vi "Spot Chessboard AR.vi"() -> ()   [LabVIEW 2020]
uses:
  g_ar_toolkit.feature_detection/Chessboard Corner Info.ctl
  g_ar_toolkit.common/Object Point (Float).ctl
  g_ar_toolkit.ar/Camera Parameters.ctl
  g_ar_toolkit.ar/Camera Matrix.ctl
  g_ar_toolkit.ar/Camera Distortion Coefficients.ctl
  g_ar_toolkit.common/Image Size (Integer).ctl
  g_ar_toolkit.ar/Point Correspondence Set.ctl
  g_ar_toolkit.common/Image Point (Float).ctl
  g_ar_toolkit.image/Image Read Size.ctl
  g_ar_toolkit.image/CreateEmptyImageGreyscale.vi
  g_ar_toolkit.image/CreateEmptyImageARGB.vi
  g_ar_toolkit.image/ReadImageFileARGB.vi
  g_ar_toolkit.feature_detection/FindChessboardCornersGreyscale.vi
  g_ar_toolkit.ar/SolvePnP-Iterative.vi
  g_ar_toolkit.image/CopyPixmapToImageFlattenMaskARGB.vi
  g_ar_toolkit.image/MaskFromColour.vi
  g_ar_toolkit.image/BitwiseNOTGreyscale.vi
  g_ar_toolkit.image/InsertImageGreyscaleMaskARGB.vi
  g_ar_toolkit.image/DrawImageToPictureGreyscale.vi
  g_ar_toolkit.image/DrawImageToPictureARGB.vi
  g_ar_toolkit.ar/Create Mesh form Verticies.vi
  g_ar_toolkit.ar/Apply Material Information.vi
  g_ar_toolkit.image/CreateEmptyImageGreyscale.vi/6598b9e0-8a08-46f5-91fd-ca1b87217137.vi
  g_ar_toolkit.image/CreateEmptyImageARGB.vi/3321fa97-f432-4e1e-8db9-a0df79aed21b.vi
  g_ar_toolkit.image/ReadImageFileARGB.vi/2358f293-6357-4b7a-bec3-c4e4d03be6e5.vi
  g_ar_toolkit.image/ARGBExtractChannel.vi
  g_ar_toolkit.feature_detection/FindChessboardCornersGreyscale.vi/ca99938f-1423-42fb-b653-ffd1f73e2bb5.vi
  g_ar_toolkit.ar/SolvePnPCore.vi
  g_ar_toolkit.ar/Rodrigues.vi
  g_ar_toolkit.ar/RodriguesRVecToRMat.vi
  <vilib>/Analysis/baseanly.llb/A x B.vi
  <vilib>/Analysis/baseanly.llb/Real A x B.vi
  g_ar_toolkit.image/CopyPixmapToImageFlattenMaskARGB.vi/80b1166a-8c06-443b-b271-eb6a715622f7.vi
  g_ar_toolkit.image/MaskFromColour.vi/5701baee-35e2-4306-9a77-a9fdbb5b3a7f.vi
  g_ar_toolkit.image/BitwiseNOTGreyscale.vi/f9ee80d6-438b-4cfb-91f1-04b98ac80474.vi
  g_ar_toolkit.image/InsertImageGreyscaleMaskARGB.vi/5e3288c8-ee88-4cfe-89cf-31ceca475f5a.vi
  g_ar_toolkit.image/DrawImageToPictureGreyscale.vi/9ae995ca-ccda-485c-89ac-02736fde3e8e.vi
  g_ar_toolkit.image/DrawImageToPictureARGB.vi/8cd07b1b-062e-4fe4-9e87-2eb3dc89fe0e.vi
  g_ar_toolkit.image/FixPixmap.vi
  g_ar_toolkit.image/Default8bitColourMap.vi
  <vilib>/Utility/error.llb/Error Cluster From Error Code.vi
  <vilib>/string/Create NI GUID.vi
  <vilib>/picture/3D Picture Control/Geometries/Create Mesh.vi
  <vilib>/picture/3D Picture Control/Object/Create Object (drawable).vi
  <vilib>/picture/3D Picture Control/Object/Set Material.vi
  <vilib>/Utility/libraryn.llb/Get File Extension.vi
  <vilib>/picture/jpeg.llb/Read JPEG File.vi
  <vilib>/picture/3D Picture Control/Helpers/Apply Texture.vi
  <vilib>/picture/3D Picture Control/Helpers/Apply Texture (no reference).vi
  <vilib>/picture/png.llb/Read PNG File.vi
  <vilib>/picture/bmp.llb/Read BMP File.vi
  <vilib>/picture/3D Picture Control/Object/Create Object (name).vi
  <vilib>/picture/3D Picture Control/Object/Add Object (no reference).vi
  <vilib>/picture/3D Picture Control/Object/Add Object (reference).vi
  g_ar_toolkit.image/ARGBColourToU32.vi
  g_ar_toolkit.common/Termination Criteria/Get Values.vi
  <vilib>/Analysis/Matrix/Numeric/Conversions/Array To Matrix.vi
  <vilib>/Analysis/Matrix/Numeric/Conversions/Array To Matrix - RA2.vi
  g_ar_toolkit.common/Termination Criteria/Termination Criteria.lvclass
  g_ar_toolkit.feature_detection/g_ar_toolkit.feature_detection.lvlib
  g_ar_toolkit.image/g_ar_toolkit.image.lvlib
  g_ar_toolkit.common/g_ar_toolkit.common.lvlib
  g_ar_toolkit.ar/g_ar_toolkit.ar.lvlib
  <vilib>/picture/3D Picture Control/NI_3D Picture Control.lvlib
  <vilib>/Utility/miscctls.llb/LVBoundsTypeDef.ctl
panel:
  out "Results":T1(array[cluster])
  out "3D Picture":refnum<vi>(3d-picture)
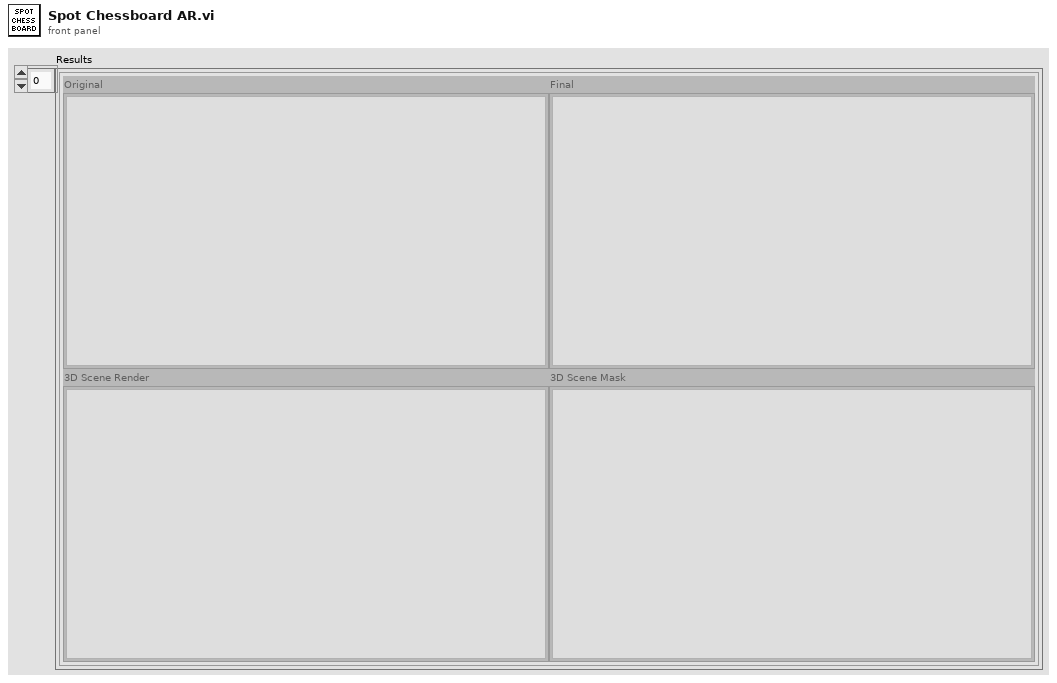
[diagram p1: front panel]
types:
  T1 = cluster{"Original":picture, "Final":picture, "3D Scene Render":picture, "3D Scene Mask":picture}[]
  T2 = typedef "g_ar_toolkit.ar.lvlib/Camera Parameters.ctl" = cluster{"Matrix":T3, "Distortion":T4, "Size":T5}
  T3 = typedef "g_ar_toolkit.ar.lvlib/Camera Matrix.ctl" = cluster{"m 0,0":dbl, "m 0,1":dbl, "m 0,2":dbl, "m 1,0":dbl, "m 1,1":dbl, "m 1,2":dbl, "m 2,0":dbl, "m 2,1":dbl, "m 2,2":dbl}
  T4 = typedef "g_ar_toolkit.ar.lvlib/Camera Distortion Coefficients.ctl" = cluster{"k1":dbl, "k2":dbl, "p1":dbl, "p2":dbl, "k3":dbl, "k4":dbl, "k5":dbl, "k6":dbl, "s1":dbl, "s2":dbl, "s3":dbl, "s4":dbl, "tau x":dbl, "tau y":dbl}
  T5 = typedef "g_ar_toolkit.common.lvlib/Image Size (Integer).ctl" = cluster{"Width":u16, "Height":u16}
  T6 = typedef "LVBoundsTypeDef.ctl" = cluster{"Width":u32, "Height":u32}
  T7 = typedef "g_ar_toolkit.common.lvlib/Object Point (Float).ctl" = cluster{"x":dbl, "y":dbl, "z":dbl}
  T8 = typedef "g_ar_toolkit.feature_detection.lvlib/Chessboard Corner Info.ctl" = cluster{"Points Per Row":u8, "Points Per Col":u8}
  T9 = cluster{"Points Per Row":i32, "Points Per Col":i32}
  T10 = cluster{"Points Per Row":dbl, "Points Per Col":dbl}
  T11 = typedef "g_ar_toolkit.image.lvlib/Image Read Size.ctl" = enum8{"FULL_SIZE", "REDUCED_2", "REDUCED_4", "REDUCED_8"}
  T12 = typedef "g_ar_toolkit.ar.lvlib/Point Correspondence Set.ctl" = cluster{"Object Points":T7[], "Image Points":T13[]}
  T13 = typedef "g_ar_toolkit.common.lvlib/Image Point (Float).ctl" = cluster{"x":dbl, "y":dbl}
  T14 = typedef "g_ar_toolkit.ar.lvlib/Pose.ctl" = cluster{"rvec":T15, "tvec":T16}
  T15 = typedef "g_ar_toolkit.ar.lvlib/rvec.ctl" = cluster{"v0":dbl, "v1":dbl, "v2":dbl}
  T16 = typedef "g_ar_toolkit.ar.lvlib/tvec.ctl" = cluster{"x":dbl, "y":dbl, "z":dbl}
  T17 = typedef "NI_Matrix.lvlib/RealMatrix.ctl" = dbl[][]
  T18 = typedef "imagedata.ctl" = cluster{"image type":i32, "image depth":i32, "image":u8[], "mask":u8[], "colors":u32[], "Rectangle":cluster{"left":i16, "top":i16, "right":i16, "bottom":i16}}
  T19 = cluster{"Picture":picture, "Picture":picture, "Picture":picture, "Picture":picture}
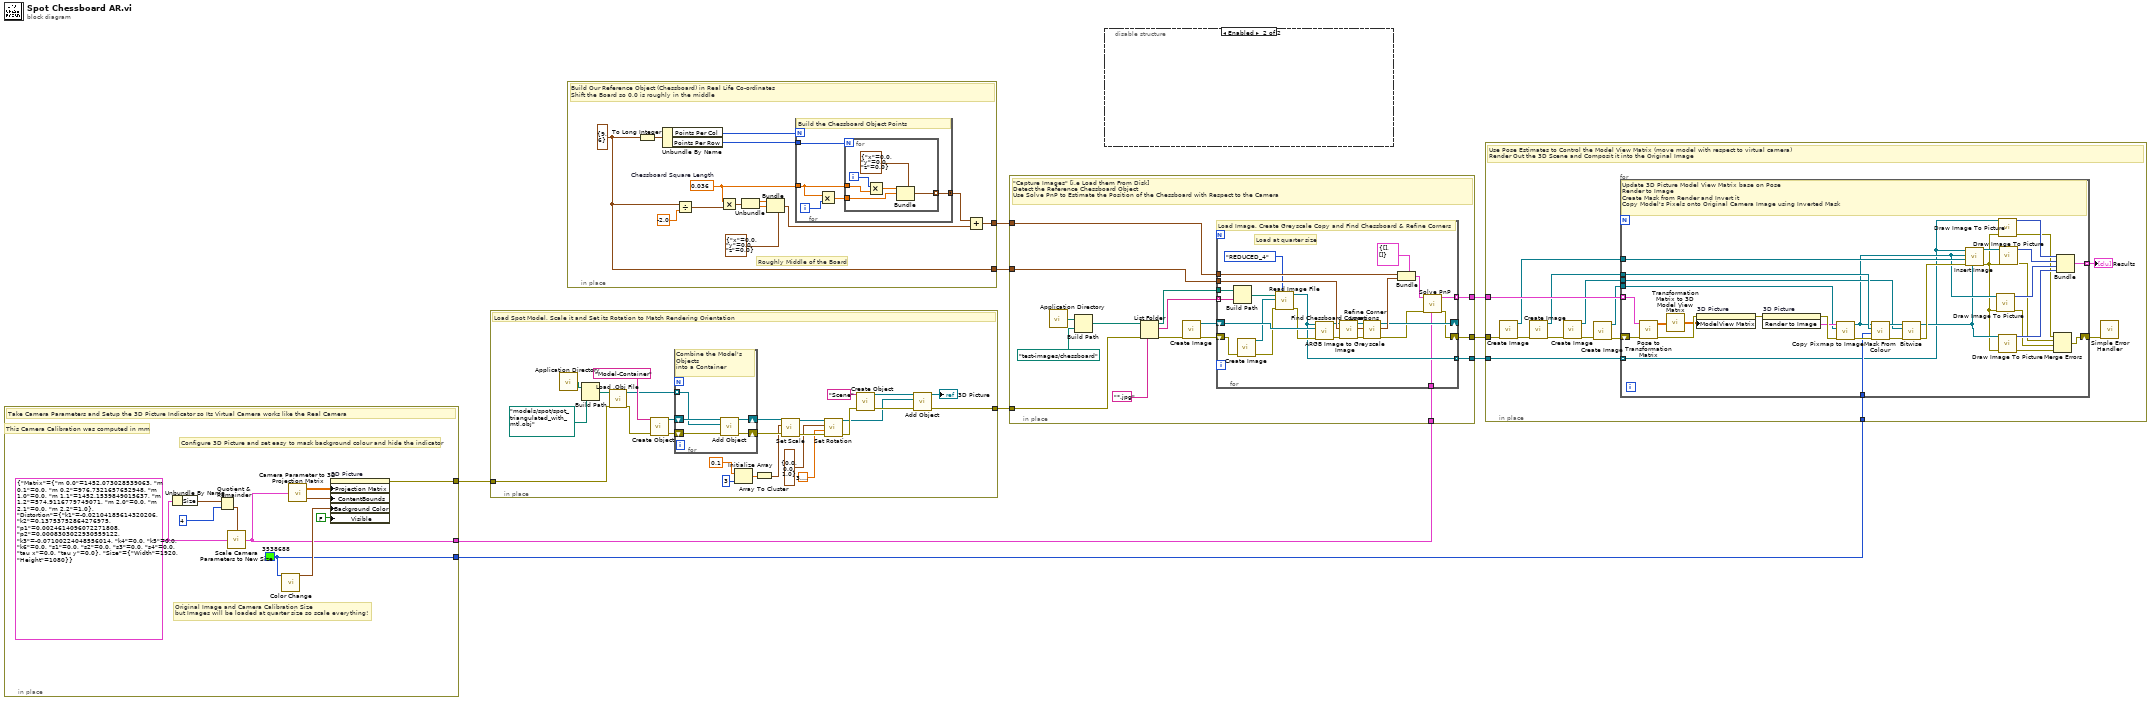
[diagram p0: block diagram]
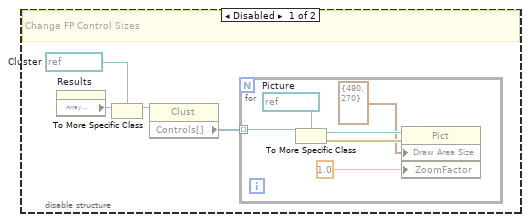
[diagram p2: hidden frame]
diagram:
  n1 = in-place {
    in-place-border: [w20] -> w8
    in-place-border: [w16] -> w5
    in-place-border: [w18] -> w3
    w18 = u32 3538688 ("Color")
    w12 = T2 {"Matrix"={"m 0,0"=1452.073028539063, "m 0,1"=0.0, "m 0,2"=976.7321657652948, "m 1,0"=0.0, "m 1,1"=1452.1539849015637, "m 1,2"=574.9116779749071, "m 2,0"=0.0, "m 2,1"=0.0, "m 2,2"=1.0}, "Distortion"={"k1"=-0.02104185614320206, "k2"=0.13753752864276975, "p1"=0.0024614096072271808, "p2"=0.0008303022930559122, "k3"=-0.07100224048556014, "k4"=0.0, "k5"=0.0, "k6"=0.0, "s1"=0.0, "s2"=0.0, "s3"=0.0, "s4"=0.0, "tau x"=0.0, "tau y"=0.0}, "Size"={"Width"=1920, "Height"=1080}} ("Camera Parameters")
    # "Original Image and Camera Calibration Size \nbut Images will be loaded at quarter size so scale everything!"
    # "Configure 3D Picture and set easy to mask background colour and hide the indicator"
    # "This Camera Calibration was computed in mm"
    # "Take Camera Parameters and Setup the 3D Picture Indicator so Its Virtual Camera works like the Real Camera"
    n2 = Unbundle By Name(w12) -> ("Size"=w11:T5)
    n3 = Quotient & Remainder(x=w11, y=u16 4) -> (floor(x/y)=w10:T5)  [unwired: 1 out]
    n4 = call "Scale Camera Parameters to New Size.vi"("Camera Parameters"=w12, "New Size"=w10) -> ("Scaled Camera Parameters"=w16:T2)
    n5 = call <vilib>:"Color Change.vi"("Color"=w18) -> ("RGBA"=w19:cluster{"R":sgl, "G":sgl, "B":sgl, "A":sgl})  [unwired: 10 in]
    n6 = call "Camera Parameter to 3D Projection Matrix.vi"("Camera Parameters"=w16) -> ("3D-Control Projection Matrix"=w13:sgl[][], "Bounds"=w14:T6)  [unwired: 4 in]
    n7 = property on="3D Picture" class="SceneGraphDisp (strict)"("Projection Matrix"=w13, "ContentBounds"=w14, "Background Color"=w19, "Visible"=FALSE) -> (error out=w20:errorcluster)  [unwired: 2 in, 1 out]
  }
  n8 = in-place {
    in-place-border: [w41] -> w9
    in-place-border: w8 -> [w40]
    # "Load Spot Model, Scale it and Set its Rotation to Match Rendering Orientation"
    n9 = call <vilib>:"Application Directory.vi"() -> ("Application Directory"=w46:path)
    n10 = Build Path(base path=w46, name or relative path=path "models/spot/spot_triangulated_with_mtl.obj" ("Path")) -> (appended path=w45:path)
    n11 = call "Load .Obj File.vi"("error in (no error)"=w40, "Object Model Path"=w45) -> ("error out"=w38:errorcluster, "Objects"=w34:refnum<vi>[])  [unwired: 7 in, 1 out]
    n12 = call-poly <vilib>:"Create Object.vi"("error in (no error)"=w38, "Name"="Model-Container") -> ("error out"=w36:errorcluster, "Scene:New Object"=w35:refnum<vi>)  [unwired: 8 in]
    n13 = for {
      tunnel: w34 -> [w49] mode=indexing
      shift-right: [w48] -> w33
      shift-left: w35 -> [w50]
      shift-right: [w47] -> w32
      shift-left: w36 -> [w51]
      # "Combine the Model's Objects\ninto a Container"
      n14 = call-poly <vilib>:"Add Object.vi"("error in (no error)"=w51, "New Object In"=w49, "Scene Object In"=w50) -> ("error out"=w47:errorcluster, "Scene Object Out"=w48:refnum<vi>)  [unwired: 7 in]
    }
    n15 = Initialize Array(0.1, 3 ("dimension size")) -> (w28:dbl[])
    n16 = Array To Cluster(array=w28) -> (cluster=w27:cluster{"[0]":dbl, "[1]":dbl, "[2]":dbl})
    n17 = call <vilib>:"Set Scale.vi"("error in (no error)"=w32, "Scale"=w27, "Scene Object"=w33) -> ("error out"=w31:errorcluster, "Scaled Object"=w25:refnum<vi>)  [unwired: 7 in]
    n18 = call <vilib>:"Set Rotation.vi"("error in (no error)"=w31, "Angle"=3.141592653589793, "Axis"=cluster{"X":sgl, "Y":sgl, "Z":sgl} {"X"=0.0, "Y"=0.0, "Z"=1.0}, "Scene Object"=w25) -> ("error out"=w26:errorcluster, "Rotated Scene Object"=w24:refnum<vi>)  [unwired: 6 in]
    n19 = call-poly <vilib>:"Create Object.vi"("error in (no error)"=w26, "Name"="Scene") -> ("error out"=w42:errorcluster, "Scene:New Object"=w43:refnum<vi>)  [unwired: 8 in]
    n20 = call-poly <vilib>:"Add Object.vi"("error in (no error)"=w42, "New Object In"=w24, "Scene Object In"=w43) -> ("error out"=w41:errorcluster, "Scene Object Out"=→"3D Picture":refnum<vi>)  [unwired: 6 in, 1 out]
  }
  n21 = in-place {
    in-place-border: [w61] -> w2
    in-place-border: [w53] -> w1
    w58 = 0.036  # Chessboard Square Length
    w61 = T8 {"Points Per Row"=9, "Points Per Col"=6} ("Chessboard Corners Info")
    # "Roughly Middle of the Board"
    # "Build Our Reference Object (Chessboard) in Real Life Co-ordinates\nShift the Board so 0,0 is roughly in the middle"
    n22 = To Long Integer(number=w61) -> (32bit integer=w62:T9)
    n23 = Unbundle By Name(w62) -> ("Points Per Col"=w65:i32, "Points Per Row"=w64:i32)
    n24 = Divide(x=w61, y=-2.0) -> (x/y=w59:T10)
    n25 = Multiply(x=w58, y=w59) -> (x*y=w57:T10)
    n26 = Unbundle(w57) -> ("Points Per Row"=w56:dbl, "Points Per Col"=w54:dbl)
    n27 = Bundle(cluster=T7 {"x"=0.0, "y"=0.0, "z"=0.0} ("Object Point"), "x"=w56, "y"=w54) -> (w52:T7)  [unwired: 1 in]
    n28 = for {
      N: w65 -> [_]
      tunnel: w64 -> [w70]
      tunnel: w58 -> [w68]
      tunnel: [w66] -> w63 mode=concatenating
      i -> [w69]
      # "Build the Chessboard Object Points"
      n29 = Multiply(x=w68, y=w69) -> (x*y=w67:dbl)
      n30 = for {
        N: w70 -> [_]
        tunnel: w68 -> [w76]
        tunnel: w67 -> [w72]
        tunnel: [w71] -> w66 mode=indexing
        i -> [w75]
        n31 = Multiply(x=w75, y=w76) -> (x*y=w73:dbl)
        n32 = Bundle(cluster=T7 {"x"=0.0, "y"=0.0, "z"=0.0} ("Object Point"), "x"=w73, "y"=w72) -> (w71:T7)  [unwired: 1 in]
      }
    }
    n33 = Add(x=w63, y=w52) -> (x+y=w53:T7[])
  }
  n34 = in-place {
    in-place-border: w9 -> [w83]
    in-place-border: [w82] -> w7
    in-place-border: [w81] -> w6
    in-place-border: w5 -> [w80]
    in-place-border: [w79] -> w4
    in-place-border: w2 -> [w78]
    in-place-border: w1 -> [w77]
    # "\"Capture Images\" [i.e Load them From Disk]\nDetect the Reference Chessboard Object\nUse Solve PnP to Estimate the Position of the Chessboard with Respect to the Camera"
    n35 = call <vilib>:"Application Directory.vi"() -> ("Application Directory"=w89:path)
    n36 = Build Path(base path=w89, name or relative path=path "test-images/chessboard") -> (appended path=w87:path)
    n37 = List Folder(path=w87, pattern="*.jpg", error in=w83) -> (path out=w86:path, filenames=w84:string[], error out=w85:errorcluster)  [unwired: 1 in, 1 out]
    n38 = call-poly "Create Image.vi"("error in (no error)"=w85) -> ("error out"=w91:errorcluster, "New Greyscale Image"=w92:refnum<data-value>)  [unwired: 9 in]
    n39 = for {
      tunnel: w86 -> [w117]
      tunnel: w84 -> [w116] mode=indexing
      shift-right: [w98] -> w79
      shift-left: w91 -> [w104]
      shift-right: [w109] -> _
      shift-left: w92 -> [w108]
      tunnel: w78 -> [w114]
      tunnel: w77 -> [w113]
      tunnel: [w100] -> w81 mode=indexing
      tunnel: w80 -> [w95]
      tunnel: [w94] -> w82 mode=indexing
      # "Load at quarter size"
      # "Load Image, Create Greyscale Copy and Find Chessboard & Refine Corners"
      n40 = Build Path(base path=w117, name or relative path=w116) -> (appended path=w115:path)
      n41 = call-poly "Create Image.vi"("error in (no error)"=w104) -> ("error out"=w103:errorcluster, "New ARGB Image"=w102:refnum<data-value>)  [unwired: 9 in]
      n42 = call-poly "Read Image File.vi"("Image Read Size (Default: FULL_SIZE)"=Image_Read_Size."REDUCED_4", "error in (no error)"=w103, "ARGB Image Destination"=w102, "Filepath"=w115) -> ("error out"=w101:errorcluster, "ARGB Image Destination (duplicate)"=w100:refnum<data-value>)  [unwired: 6 in]
      n43 = call "ARGB Image to Greyscale Image.vi"("error in (no error)"=w101, "Greyscale Image Destination"=w108, "ARGB Image Source"=w100) -> ("error out"=w105:errorcluster, "Greyscale Image Destination (Duplicate)"=w107:refnum<data-value>)  [unwired: 7 in]
      n44 = call-poly "Find Chessboard Corners.vi"("error in (no error)"=w105, "Chessboard Corners Info"=w114, "Greyscale Image"=w107) -> ("error out"=w112:errorcluster, "Points"=w111:T13[], "Greyscale Image (Duplicate)"=w106:refnum<data-value>)  [unwired: 6 in]
      n45 = call "Refine Corner Locations.vi"("error in (no error)"=w112, "Points in"=w111, "Greyscale Image"=w106) -> ("error out"=w99:errorcluster, "Points out"=w110:T13[], "Greyscale Image (Duplicate)"=w109:refnum<data-value>)  [unwired: 6 in]
      n46 = Bundle(cluster=T12 {"Object Points"=[], "Image Points"=[]} ("Point Correspondence Set"), "Object Points"=w113, "Image Points"=w110) -> (w96:T12)
      n47 = call-poly "Solve PnP.vi"("Camera Parameters"=w95, "error in (no error)"=w99, "Point Correspondence Set"=w96) -> ("error out"=w98:errorcluster, "Pose"=w94:T14)  [unwired: 7 in]
    }
  }
  n48 = disable-structure shown="Enabled" {
    frame Disabled {
      w119 = refnum<vi> refnum  # Cluster
      # "Change FP Control Sizes"
      n49 = property on="Results" class="Arr (strict)"() -> ("Array Element"=w121:refnum<vi>)  [unwired: 2 in, 2 out]
      n50 = To More Specific Class(target class=w119, reference=w121) -> (specific class reference=w120:refnum<vi>)  [unwired: 1 in, 1 out]
      n51 = property class="Clust"(reference=w120) -> ("Controls[]"=w118:refnum<vi>[])  [unwired: 1 in, 2 out]
      n52 = for {
        tunnel: w118 -> [w127] mode=indexing
        w126 = refnum<vi> refnum  # Picture
        n53 = To More Specific Class(target class=w126, reference=w127) -> (specific class reference=w125:refnum<vi>, error out=w124:errorcluster)  [unwired: 1 in]
        n54 = property class="Pict"(reference=w125, error in=w124, "Draw Area Size"=T6 {"Width"=480, "Height"=270}, "ZoomFactor"=sgl 1.0 ("Zoom Factor")) -> ()  [unwired: 2 out]
      }
    }
    frame Enabled {
    }
  }
  n55 = in-place {
    in-place-border: w7 -> [w141]
    in-place-border: w6 -> [w140]
    in-place-border: w4 -> [w139]
    in-place-border: w3 -> [w132]
    # "Use Pose Estimates to Control the Model View Matrix (move model with respect to virtual camera)\nRender Out the 3D Scene and Composit it into the Original Image"
    n56 = call-poly "Create Image.vi"("error in (no error)"=w139) -> ("error out"=w135:errorcluster, "New ARGB Image"=w134:refnum<data-value>)  [unwired: 9 in]
    n57 = call-poly "Create Image.vi"("error in (no error)"=w135) -> ("error out"=w131:errorcluster, "New Greyscale Image"=w138:refnum<data-value>)  [unwired: 9 in]
    n58 = call-poly "Create Image.vi"("error in (no error)"=w131) -> ("error out"=w130:errorcluster, "New Greyscale Image"=w129:refnum<data-value>)  [unwired: 9 in]
    n59 = call-poly "Create Image.vi"("error in (no error)"=w130) -> ("error out"=w137:errorcluster, "New ARGB Image"=w136:refnum<data-value>)  [unwired: 9 in]
    n60 = for {
      tunnel: w141 -> [w171] mode=indexing
      tunnel: w140 -> [w153] mode=indexing
      tunnel: w138 -> [w164]
      tunnel: w136 -> [w165]
      tunnel: w134 -> [w163]
      shift-right: [w143] -> w133
      shift-left: w137 -> [w170]
      tunnel: w132 -> [w160]
      tunnel: w129 -> [w156]
      tunnel: [w142] -> w128 mode=indexing
      # "Update 3D Picture Model View Matrix base on Pose\nRender to Image\nCreate Mask from Render and Invert it\nCopy Model's Pixels onto Original Camera Image using Inverted Mask"
      n61 = call "Pose to Transformation Matrix.vi"("error in (no error)"=w170, "Pose"=w171) -> ("error out"=w172:errorcluster, "Transformation Matrix"=w161:T17)  [unwired: 8 in]
      n62 = call "Transformation Matrix to 3D Model View Matrix.vi"("Transformation Matrix"=w161) -> ("3D-Control Model Matrix"=w169:T17)
      n63 = property on="3D Picture" class="SceneGraphDisp (strict)"(error in=w172, "ModelView Matrix"=w169) -> (error out=w168:errorcluster)  [unwired: 1 in, 1 out]
      n64 = invoke on="3D Picture" class="SceneGraphDisp (strict)" method="Render to Image"(error in=w168) -> (error out=w173:errorcluster, "Get Image"=w167:T18)  [unwired: 2 in, 1 out]
      n65 = call-poly "Copy Pixmap to Image.vi"("error in (no error)"=w173, "ARGB Image Destination"=w165, "Pixmap Image Data"=w167) -> ("error out"=w166:errorcluster, "ARGB Image Destination (duplicate)"=w155:refnum<data-value>)  [unwired: 7 in]
      n66 = call-poly "Mask From Colour.vi"("error in (no error)"=w166, "Value"=w160, "Mask Destination"=w164, "ARGB Image Source"=w155) -> ("error out"=w158:errorcluster, "Mask Destination (duplicate)"=w159:refnum<data-value>)  [unwired: 6 in]
      n67 = call-poly "Bitwise.vi"("error in (no error)"=w158, "Greyscale Image Destination"=w156, "Greyscale Image Source"=w159) -> ("error out"=w157:errorcluster, "Greyscale Image Destination (duplicate)"=w154:refnum<data-value>)  [unwired: 7 in]
      n68 = call-poly "Insert Image.vi"("Greyscale Image Mask"=w154, "error in (no error)"=w157, "ARGB Image Destination"=w163, "ARGB Image Child"=w155, "ARGB Image Parent"=w153) -> ("error out"=w152:errorcluster, "ARGB Image Destination (duplicate)"=w162:refnum<data-value>)  [unwired: 5 in]
      n69 = call-poly "Draw Image To Picture.vi"("error in (no error)"=w152, "ARGB Image Source"=w155) -> ("error out"=w146:errorcluster, "Picture"=w149:picture)  [unwired: 8 in]
      n70 = call-poly "Draw Image To Picture.vi"("error in (no error)"=w152, "ARGB Image Source"=w153) -> ("error out"=w145:errorcluster, "Picture"=w151:picture)  [unwired: 8 in]
      n71 = call-poly "Draw Image To Picture.vi"("error in (no error)"=w152, "Greyscale Image Source"=w154) -> ("error out"=w147:errorcluster, "Picture"=w148:picture)  [unwired: 8 in]
      n72 = call-poly "Draw Image To Picture.vi"("error in (no error)"=w152, "ARGB Image Source"=w162) -> ("error out"=w144:errorcluster, "Picture"=w150:picture)  [unwired: 8 in]
      n73 = Merge Errors(w145, w144, w146, w147) -> (w143:errorcluster)
      n74 = Bundle("Picture"=w151, "Picture"=w150, "Picture"=w149, "Picture"=w148) -> (w142:T19)  [unwired: 1 in]
    }
    "Results" <- w128
    n75 = call <vilib>:"Simple Error Handler.vi"("error in (no error)"=w133) -> ()  [unwired: 4 in, 5 out]
  }
